vi "GasflaschenHeader_Kopfzeile_entfernen.vi"(11 "Array (Eingang)":string[][](array[string])) -> (3 "Array (Ausgang)":string[][](array[string]))   [LabVIEW 2020, in "System Einstellungen V2.lvlib"]
uses:
  System Einstellungen V2.lvlib
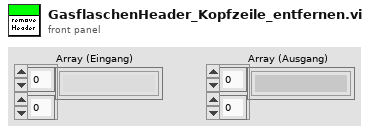
[diagram p1: front panel]
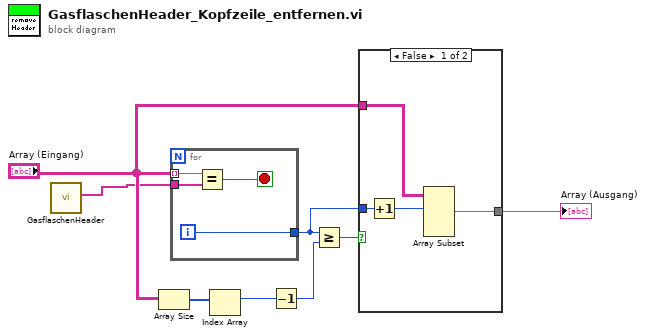
[diagram p0: block diagram]
diagram:
  n1 = call "GasflaschenHeader.vi"() -> ("Trennlinie"=w2:string[])  [unwired: 10 in, 1 out]
  n2 = Array Size(array="Array (Eingang)") -> (size(s)=w8:i32[])
  n3 = for {
    tunnel: "Array (Eingang)" -> [w12] mode=indexing
    tunnel: w2 -> [w11]
    tunnel: [w9] -> w1
    i -> [w9]
    stop <- w10 stop-if-true
    n4 = Equal?(x=w12, y=w11) -> (x = y?=w10:bool)
  }
  n5 = Index Array(array=w8) -> (element=w5:i32)  [unwired: 1 in]
  n6 = Decrement(x=w5) -> (x-1=w7:i32)
  n7 = Greater Or Equal?(x=w1, y=w7) -> (x >= y?=w6:bool)
  n8 = case shown="False" w6 {
    tunnel: "Array (Eingang)" -> [w16 w17]
    tunnel: w1 -> [w15 _]
    tunnel: [w14 w17] -> w3
    frame False {
      n9 = Increment(x=w15) -> (x+1=w13:i32)
      n10 = Array Subset(array=w16, index (row)=w13) -> (w14:string[][])  [unwired: 3 in]
    }
    frame True {
    }
  }
  "Array (Ausgang)" <- w3
